vi "Pre Launch Init.vi"(11 "Test Actor in":refnum<class "Test Actor.lvclass">) -> (0 "error out":errorcluster, 3 "Test Actor out":refnum<class "Test Actor.lvclass">)   [LabVIEW 2020, in "Test.lvlib" / "Test Actor.lvclass"]
doc: "(<B>Filename</B>: Actor Framework.lvlib:Actor.lvclass:Pre Launch Init.vi)\n\nDefines behavior that occurs after the Launch Nested Actor method is invoked but before the actor's Actor Core method begins running.\n\nBy default, this method does nothing. A descendant class may override it to define behavior."
uses:
  Test Actor.lvclass
  Test Actor.lvclass/Test Actor.ctl
  PPL/HDH.Actor Framework.Core.Sequencer.lvlibp/Sequencer/Sequencer.lvclass
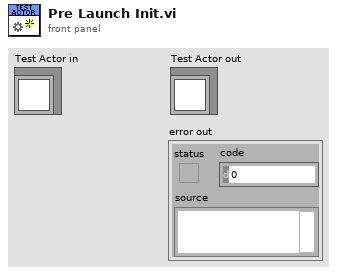
[diagram p1: front panel]
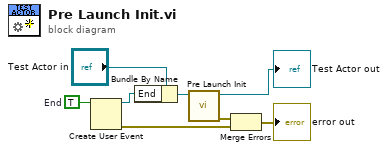
[diagram p0: block diagram]
diagram:
  w5 = TRUE  # End
  n1 = Create User Event(user event datatype=w5) -> (user event=w3:refnum<user-event>, error out=w1:errorcluster)  [unwired: 1 in]
  n2 = Bundle By Name(cluster="Test Actor in", "End"=w3) -> (w4:refnum<class "Test Actor.lvclass">)
  n3 = call-parent "Pre Launch Init.vi"("Sequencer in"=w4) -> ("error out"=w8:errorcluster, "Sequencer out"=→"Test Actor out":refnum<class "Test Actor.lvclass">)  [unwired: 9 in]
  n4 = Merge Errors(w8, w1) -> (→"error out":errorcluster)
